vi "BPIM Sim ID to TestSet.vi"(11 "SimID":u32) -> (2 "PIM System":T1 {"Modules"."DevID" format="%.0x"}, 3 "Test Set Definition":T5={"General"={"ID"=0, "Model"="", "Dual Port?"=FALSE, "Options"="", "Options"={"E"=FALSE, "K"=FALSE, "H"=FALSE, "W"=FALSE, "F"=FALSE}, "Cal File"=path ""}, "Receiver"={"Fstart, MHz"=0.0, "Fstop MHz"=0.0, "Fstep MHz"=0.0, "IF, MHz"=0.0}, "RX Band"={"Fstart, MHz"=0.0, "Fstop MHz"=0.0}, "TX 1"={"Fstart, MHz"=0.0, "Fstop MHz"=0.0, "Pmax, dBm"=0.0, "Pstep, dB"=0.0}, "TX 2"={"Fstart, MHz"=0.0, "Fstop MHz"=0.0, "Pmax, dBm"=0.0, "Pstep, dB"=0.0}, "Low-side?"=TRUE})   [LabVIEW 2011]
uses:
  HW IO/Test Set Definition.ctl
  WebEngine/LIB/PIM System Definition.ctl
  WebEngine/LIB/MODULES/ModuleDef.ctl
  WebEngine/LIB/MODULES/Module_Types.ctl
  WebEngine/LIB/ProcLoops/BPIM.Analyzer.Series.ctl
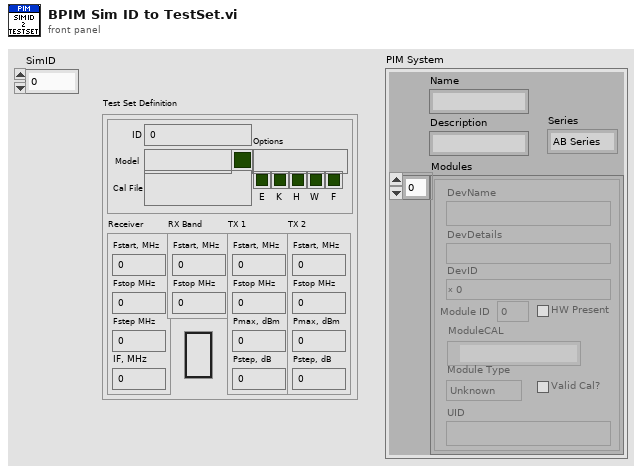
[diagram p1: front panel]
types:
  T1 = typedef "PIM System Definition.ctl" = cluster{"Name":string, "Description":string, "Modules":T2[], "Series":T4}
  T2 = typedef "ModuleDef.ctl" = cluster{"DevName":string, "DevDetails":string, "DevID":u32, "HW Present":bool, "Module ID":u16, "ModuleCAL":path, "Module Type":T3, "Valid Cal?":bool, "UID":string}
  T3 = typedef "Module_Types.ctl" = enum16{"Unknown", "RF Module", "PA Module", "TR Module", "FE Module", "SW Module"}
  T4 = typedef "BPIM.Analyzer.Series.ctl" = enum16{"AB Series", "D Series", "E Series", "Simulator"}
  T5 = typedef "Test Set Definition.ctl" = cluster{"General":cluster{"ID":u32, "Model":string, "Dual Port?":bool, "Options":string, "Options":cluster{"E":bool, "K":bool, "H":bool, "W":bool, "F":bool}, "Cal File":path}, "Receiver":cluster{"Fstart, MHz":dbl, "Fstop MHz":dbl, "Fstep MHz":dbl, "IF, MHz":dbl}, "RX Band":cluster{"Fstart, MHz":dbl, "Fstop MHz":dbl}, "TX 1":cluster{"Fstart, MHz":dbl, "Fstop MHz":dbl, "Pmax, dBm":dbl, "Pstep, dB":dbl}, "TX 2":cluster{"Fstart, MHz":dbl, "Fstop MHz":dbl, "Pmax, dBm":dbl, "Pstep, dB":dbl}, "Low-side?":bool}
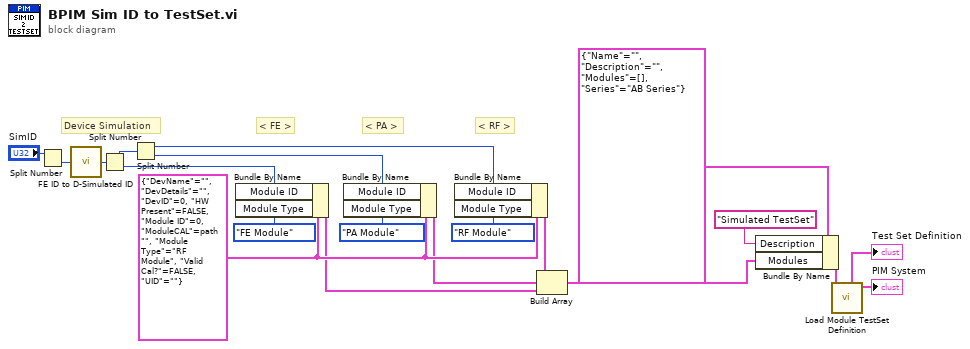
[diagram p0: block diagram]
diagram:
  w16 = T2 {"DevName"="", "DevDetails"="", "DevID"=0, "HW Present"=FALSE, "Module ID"=0, "ModuleCAL"=path "", "Module Type"=enum."RF Module", "Valid Cal?"=FALSE, "UID"=""} ("PIM Device Module")
  # "< FE >"
  # "< PA >"
  # "< RF >"
  # "Device Simulation"
  n1 = Split Number(x="SimID") -> (lo(x)=w2:u16)  [unwired: 1 out]
  n2 = call "FE ID to D-Simulated ID.vi"("B-series ID"=w2) -> ("Config 'D' ID"=w1:i32)  [unwired: 14 in]
  n3 = Split Number(x=w1) -> (hi(x)=w20:u16, lo(x)=w7:u16)
  n4 = Split Number(x=w20) -> (hi(x)=w6:u8, lo(x)=w8:u8)
  n5 = Bundle By Name(cluster=w16, "Module ID"=w7, "Module Type"=Module_Types."FE Module") -> (w13:T2)
  n6 = Bundle By Name(cluster=w16, "Module ID"=w8, "Module Type"=Module_Types."PA Module") -> (w14:T2)
  n7 = Bundle By Name(cluster=w16, "Module ID"=w6, "Module Type"=Module_Types."RF Module") -> (w15:T2)
  n8 = Build Array(w15, w14, w13) -> (w10:T2[])
  n9 = Bundle By Name(cluster=T1 {"Name"="", "Description"="", "Modules"=[], "Series"=enum."AB Series"} ("PIM System"), "Description"="Simulated TestSet", "Modules"=w10) -> (w11:T1)
  n10 = call "Load Module TestSet Definition.vi"("PIM System"=w11) -> ("PIM System out"=→"PIM System":T1, "Test Set Definition"=→"Test Set Definition":T5)  [unwired: 8 in, 1 out]
